vi "Alicat Server.vi"(0 "DVR In":refnum<data-value>) -> (14 "DVR out":refnum<data-value>)   [LabVIEW 2015]
uses:
  Data/Nicholas Data.lvclass
  Devices/Alicat/Session Based/Alicat Device.lvclass
  Reusable/Session APIs/Serial/Serial Session.lvclass
  <vilib>/Platform/TimedLoop/XDataNode/timing_clust.ctl
  <vilib>/Platform/TimedLoop/XDataNode/nitl_modes.ctl
  <vilib>/Platform/TimedLoop/XDataNode/wakeup.ctl
  Reusable/Session APIs/File Access/Config Data/Config Data.lvclass
  Reusable/Session Log/System Log.lvclass
  Reusable/Session APIs/File Access/Config Data/Config Data.lvclass/Config Data.ctl
  Reusable/Session Log/System Log.lvclass/System Log.ctl
  Reusable/Session APIs/File Access/Config Data/Config Session.ctl
  Reusable/Session APIs/Text Communication/Text Device Session.lvclass/Text Device Session.ctl
  Devices/Alicat/Session Based/Alicat Device.lvclass/Alicat Device.ctl
  Devices/Configurable Device/Configurable Device.lvclass/Configurable Device.ctl
  Devices/Alicat/Session Based/Data/Alicat Data.lvclass
  Data/Nicholas Data.lvclass/Nicholas Data.ctl
  Reusable/Session APIs/Text Communication/Write hSysLog.vi
  Devices/Alicat/Session Based/Accessors/Write ID.vi
  Devices/Configurable Device/Write Handle.vi
  Devices/Alicat/Session Based/Accessors/Write Session Handle.vi
  Devices/Alicat/Session Based/Accessors/Read Qsp.vi
  Data/Write Alicat Data.vi
  Reusable/Session APIs/File Access/Config Data/Accessors/Write Cfg Path.vi
  Reusable/Session Log/Accessors/Write Main Path.vi
  <vilib>/Platform/TimedLoop/XDataNode/XDataNode.xnode
  <userlib>/_Session Fwk/Session - Root.lvclass
  <vilib>/Platform/TimedLoop/XDataNode/XDNodeRunTimeDep.lvlib
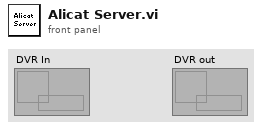
[diagram p1: front panel]
types:
  T1 = typedef "Config Data.lvclass/Config Session.ctl" = refnum<data-value>
  T2 = typedef "Session - Root.lvclass/Session Handle.ctl" = refnum<data-value>
  T3 = typedef "XDNodeRunTimeDep.lvlib/timing_clust.ctl" = cluster{"Expected End [f-1]":u64, "Actual End [f-1]":u64, "Finished Late? [f-1]":bool, "Expected End [i-1]":u64, "Actual End [i-1]":u64, "Finished Late? [i-1]":bool, "Expected Start [i]":u64, "Actual Start [i]":u64, "Expected Start [f]":u64, "Actual Start [f]":u64, "Source Name":string, "Structure Name":string, "Period":i64, "Deadline":i64, "Offset":i64, "Start":i64, "Priority":i32, "Timeout":i32, "Mode":T4, "Wakeup Reason":T5, "Error":errorcluster, "Source Type":string, "Secondary Source Type":string, "Global End Time":u64, "Global Start Time":u64, "Frame Duration":u64, "Iteration Duration":u64, "Assigned CPU":i32, "I/O Scan Engine Mode":u32}
  T4 = typedef "XDNodeRunTimeDep.lvlib/nitl_modes.ctl" = enum32{"No Change", "Process missed periods, maintain original phase", "Discard missed periods, maintain original phase", "Process missed periods, ignore original phase", "Discard missed periods, ignore original phase"}
  T5 = typedef "XDNodeRunTimeDep.lvlib/wakeup.ctl" = enum32{"Normal", "Aborted", "Asynchronous wakeup", "Timing source error", "Timed loop error", "Timeout"}
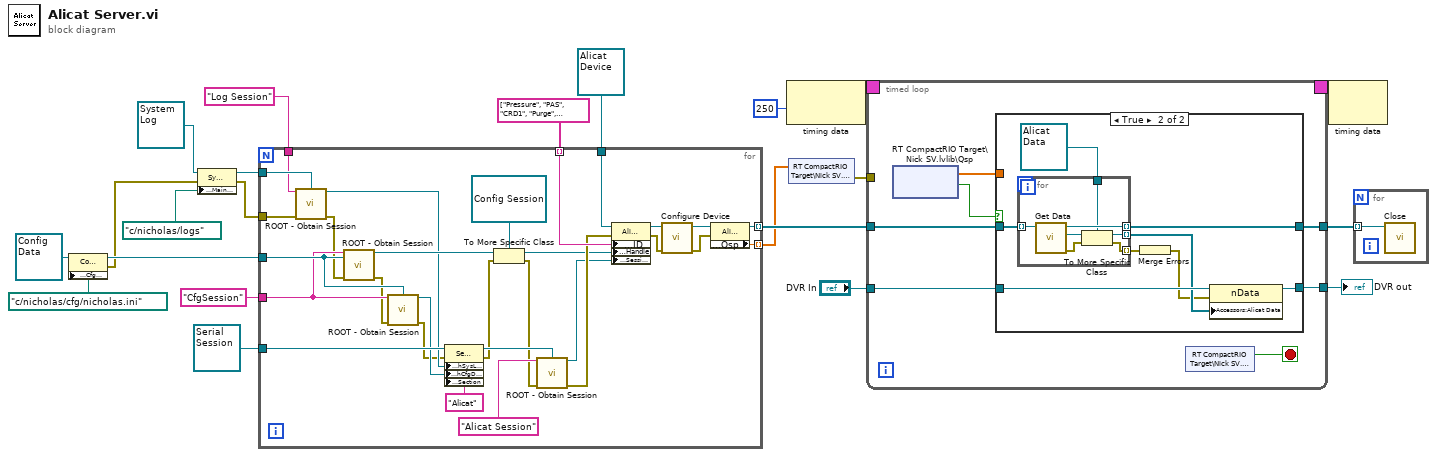
[diagram p0: block diagram]
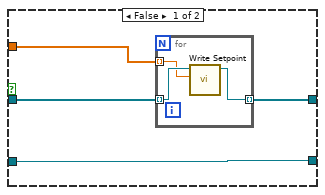
[diagram p2: hidden frame]
diagram:
  n1 = property class="Config Data"(reference=refnum<class "Config Data.lvclass"> refnum ("Config Data"), "Accessors:Cfg Path"=path "c:/nicholas/cfg/nicholas.ini" ("Cfg Path")) -> (reference out=w16:refnum<class "Config Data.lvclass">, error out=w4:errorcluster)  [unwired: 1 in]
  n2 = property class="Sys Log"(reference=refnum<class "System Log.lvclass"> refnum ("Sys Log"), error in=w4, "Accessors:Main Path"=path "c:/nicholas/logs" ("Main Path")) -> (reference out=w19:refnum<class "System Log.lvclass">, error out=w5:errorcluster)
  n3 = for {
    tunnel: refnum<class "Alicat Device.lvclass"> refnum ("Alicat Device") -> [w51]
    tunnel: w16 -> [w40]
    tunnel: "CfgSession" ("Session Name ()") -> [w39]
    tunnel: w19 -> [w50]
    tunnel: refnum<class "Serial Session.lvclass"> refnum ("Serial Session") -> [w49]
    tunnel: string[] ["Pressure", "PAS", "CRD1", "Purge", "Ozone", "AC6"] -> [w46] mode=indexing
    tunnel: [w26] -> w10 mode=indexing
    tunnel: w5 -> [w41]
    tunnel: "Log Session" ("Session Name ()") -> [w32]
    tunnel: [w24] -> w2 mode=indexing
    n4 = call <userlib>:"ROOT - Obtain Session.vi"("Session Name ()"=w32, "OBJ - Session"=w50, "error in (no error)"=w41) -> ("Session Handle"=w36:T2, "error out"=w31:errorcluster)  [unwired: 10 in, 1 out]
    n5 = call <userlib>:"ROOT - Obtain Session.vi"("Session Name ()"=w39, "OBJ - Session"=w40, "error in (no error)"=w31) -> ("Session Handle"=w38:T2, "error out"=w33:errorcluster)  [unwired: 10 in, 1 out]
    n6 = call <userlib>:"ROOT - Obtain Session.vi"("Session Name ()"=w39, "OBJ - Session"=w40, "error in (no error)"=w33) -> ("Session Handle"=w37:T2, "error out"=w30:errorcluster)  [unwired: 10 in, 1 out]
    n7 = property class="Serial Session"(reference=w49, error in=w30, "Accessors:hSysLog"=w36, "Accessors:hCfgData"=w37, "Accessors:Section"="Alicat" ("Section")) -> (reference out=w48:refnum<class "Serial Session.lvclass">, error out=w29:errorcluster)
    n8 = To More Specific Class(target class=T1 refnum ("Handle"), reference=w38, error in=w29) -> (specific class reference=w34:T1, error out=w28:errorcluster)
    n9 = call <userlib>:"ROOT - Obtain Session.vi"("Session Name ()"="Alicat Session", "OBJ - Session"=w48, "error in (no error)"=w28) -> ("Session Handle"=w35:T2, "error out"=w42:errorcluster)  [unwired: 10 in, 1 out]
    n10 = property class="Alicat Device"(reference=w51, error in=w42, "Accessors:ID"=w46, "Accessors:Handle"=w34, "Accessors:Session Handle"=w35) -> (reference out=w44:refnum<class "Alicat Device.lvclass">, error out=w43:errorcluster)
    n11 = call-dynamic "Configure Device.vi"("error in"=w43, "Alicat Device in"=w44) -> ("error out"=w25:errorcluster, "Alicat Device out"=w27:refnum<class "Alicat Device.lvclass">)  [unwired: 8 in]
    n12 = property class="Alicat Device"(reference=w27, error in=w25) -> (reference out=w26:refnum<class "Alicat Device.lvclass">, "Accessors:Qsp"=w24:dbl)  [unwired: 1 out]
  }
  n13 = node-c288(i64 250 ("Period")) -> (w22:T3)
  n14 = shared-variable "RT CompactRIO Target\\Nick SV.lvlib\\Qsp"(w2) -> (error out=w1:errorcluster)  [unwired: 1 in]
  n15 = timed-loop {
    tunnel: w10 -> [w58]
    tunnel: [w56] -> w11
    timing: w22 -> [_]
    timing-out: [_] -> w21
    tunnel: "DVR In" -> [w53]
    tunnel: [w52] -> w20
    tunnel: w1 -> [_]
    stop <- w57 stop-if-true
    n16 = shared-variable "RT CompactRIO Target\\Nick SV.lvlib\\Qsp"() -> (w54:sgl[], w55:bool)  [unwired: 2 in, 1 out]
    n17 = case shown="True" w55 {
      tunnel: w58 -> [w61 w73]
      tunnel: [w60 w72] -> w56
      tunnel: w54 -> [w62 _]
      tunnel: w53 -> [w59 w70]
      tunnel: [w59 w68] -> w52
      frame False {
        n18 = for {
          tunnel: w62 -> [w64] mode=indexing
          tunnel: w61 -> [w65] mode=indexing
          tunnel: [w63] -> w60 mode=indexing
          n19 = call "Write Setpoint.vi"("Setpoint"=w64, "Alicat Device in"=w65) -> ("Alicat Device out"=w63:refnum<class "Alicat Device.lvclass">)  [unwired: 7 in, 2 out]
        }
      }
      frame True {
        n20 = for {
          tunnel: w73 -> [w80] mode=indexing
          tunnel: [w79] -> w72 mode=indexing
          tunnel: refnum<class "Alicat Data.lvclass"> refnum ("Alicat Data") -> [w78]
          tunnel: [w76] -> w69 mode=indexing
          tunnel: [w74] -> w67 mode=indexing
          n21 = call-dynamic "Get Data.vi"("Cfg Dev in"=w80) -> ("error out"=w75:errorcluster, "DataOut"=w77:refnum<class "Data.lvclass">, "Cfg Dev out"=w79:refnum<class "Alicat Device.lvclass">)  [unwired: 8 in]
          n22 = To More Specific Class(target class=w78, reference=w77, error in=w75) -> (specific class reference=w76:refnum<class "Alicat Data.lvclass">, error out=w74:errorcluster)
        }
        n23 = Merge Errors(w67) -> (w66:errorcluster)
        n24 = property class="nData"(reference=w70, error in=w66, "Accessors:Alicat Data"=w69) -> (reference out=w68:refnum<data-value>)  [unwired: 1 out]
      }
    }
    n25 = shared-variable "RT CompactRIO Target\\Nick SV.lvlib\\Stop"() -> (w57:bool)  [unwired: 1 in, 1 out]
  }
  "DVR out" <- w20
  n26 = node-c288(w21) -> ()  [unwired: 1 out]
  n27 = for {
    tunnel: w11 -> [w83] mode=indexing
    n28 = call-dynamic "Close.vi"("Cfg Dev in"=w83) -> ()  [unwired: 9 in, 2 out]
  }
